vi "Lidar Motor Controler.vi"() -> ()   [LabVIEW 2009]
uses:
  Motor Output Global.vi
  Motor Control Global.vi
panel:
  out "number":fxp<+/-,18,1> format="%.18g"
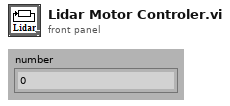
[diagram p1: front panel]
types:
  T1 = typedef "Strict Lidar Motor Control Cluster.ctl" = cluster{"Reset Encoder":bool, "Motor Enable":bool, "Choice of Control Type":enum32{"Direct Voltage Control", "Proportional Control", "PI Control", "Custom Compensator", "PID Control", "II-PID-DD Control"}, "Choice of Oscillation":enum32{"Oscillate Voltage", "Oscillate Setpoint", "No Oscillation"}, "Choice of Compensation":enum32{"None", "Computed Torque", "Mechanical Advantage", "CT & MA "}, "Choice of Error":enum32{"Gray Error", "Lidar Error", "Kent Error", "UberKent Error"}, "Units of pi rad 18b (s-fxp-1)":cluster{"Phi_B Set Point (pi rad)":fxp<+/-,18,1>, "Phi_A Set Point (pi rad)":fxp<+/-,18,1>, "Phi_Lidar Set Point (pi rad)":fxp<+/-,18,1>, "Phi_Lidar - Phi_A":fxp<+/-,18,1>, "Phi_mass-Phi_Lidar":fxp<+/-,18,1>, "Convert (enc) to (pi rad)":fxp<+/-,18,1>, "Oscillation Frequency (pi rad per 100KHz)":fxp<+/-,18,1>}, "Units of 18b (s-fxp-1) gain":cluster{"Proportional Gain":fxp<+/-,18,1>, " Integral Gain":fxp<+/-,18,1>, "Oscillation Setpoint Amplitude":fxp<+/-,18,1>, "Gravity Compensation Gain":fxp<+/-,18,1>, "Phi_B Set Point (enc) pre-gain":fxp<+/-,18,1>, "Phi_B Set Point (pi rad) pre-gain":fxp<+/-,18,1>, "Phi_A Set Point (pi rad) pre-gain":fxp<+/-,18,1>, "Phi_Lidar Set Point (pi rad) pre-gain":fxp<+/-,18,1>, "Derivative Gain":fxp<+/-,18,1>, "Double Integral Gain":fxp<+/-,18,1>, "Second Derivative Gain":fxp<+/-,18,1>}, "Units of 20b s-fxp-5 Voltage":cluster{"Oscillation Voltage Amplitude":fxp<+/-,20,5>, "Motor Voltage":fxp<+/-,20,5>}, "Units of encoder 32b uint":cluster{"Phi_B Set Point (enc)":i32, "Lidar Encoder Cap":i32}, "Debug Args":bool[], "Units of 8b int gain exponents":cluster{"Proportional Gain":i8, " Integral Gain":i8, "Oscillation Setpoint Amplitude":i8, "Gravity Compensation Gain":i8, "Phi_B Set Point (enc) pre-gain":i8, "Phi_B Set Point (pi rad) pre-gain":i8, "Phi_A Set Point (pi rad) pre-gain":i8, "Phi_Lidar Set Point (pi rad) pre-gain":i8, "Derivative Gain":i8, "Double Integral Gain":i8, "Second Derivative Gain":i8}}
  T2 = cluster{"Debug Args[0]":bool, "Debug Args[1]":bool, "Debug Args[2]":bool, "Debug Args[3]":bool, "Debug Args[4]":bool, "Debug Args[5]":bool, "Debug Args[6]":bool, "Debug Args[7]":bool, "Debug Args[8]":bool}
  T3 = typedef "Strict Lidar Motor Indicator Cluster.ctl" = cluster{"Phi_A":fxp<+/-,18,1>, "Phi_B":fxp<+/-,18,1>, "Output Voltage":fxp<+/-,20,5>, "Phi_Lidar":fxp<+/-,18,1>, "Phi_Mass":fxp<+/-,18,1>, "MA":fxp<+/-,18,1>, "Base Output":fxp<+/-,18,1>, "Error":fxp<+/-,18,1>, "Low Enc":i32, "High Enc":i32}
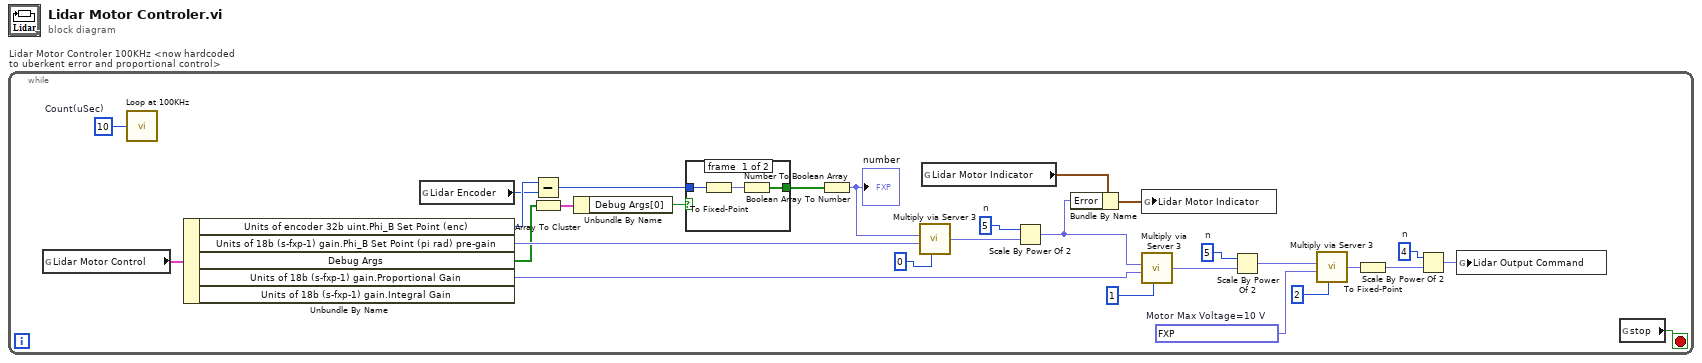
[diagram p0: block diagram]
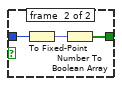
[diagram p2: hidden frame]
diagram:
  n1 = while "Lidar Motor Controler 100KHz <now hardcoded to uberkent error and proportional control>" {
    stop <- w29 stop-if-true
    w2 = 4  # n
    w5 = fxp<+/-,18,1> 0.625  # Motor Max Voltage=10 V
    w13 = 5  # n
    w14 = 5  # n
    w28 = u32 10  # Count(uSec)
    n2 = global read "Motor Control Global.vi" "Lidar Motor Control"() -> (w23:T1)
    n3 = call "Loop at 100KHz"("Count(uSec)"=w28) -> ()  [unwired: 1 out]
    n4 = Unbundle By Name(w23) -> ("Units of encoder 32b uint.Phi_B Set Point (enc)"=w22:i32, "Units of 18b (s-fxp-1) gain.Phi_B Set Point (pi rad) pre-gain"=w20:fxp<+/-,18,1>, "Debug Args"=w19:bool[], "Units of 18b (s-fxp-1) gain.Proportional Gain"=w16:fxp<+/-,18,1>)  [unwired: 1 out]
    n5 = global read "Motor Control Global.vi" "Lidar Encoder"() -> (w21:i32)
    n6 = Subtract(x=w22, y=w21) -> (x-y=w8:i32)
    n7 = Array To Cluster(array=w19) -> (cluster=w18:T2)
    n8 = Unbundle By Name(w18) -> ("Debug Args[0]"=w17:bool)
    n9 = case shown="True" w17 {
      tunnel: [w31 w35] -> w27
      tunnel: w8 -> [w30 w33]
      frame #0 {
        n10 = To Fixed-Point(number=w30) -> (fixed-point=w32:fxp<+/-,18,18>)  [unwired: 1 in]
        n11 = Number To Boolean Array(number=w32) -> (Boolean array=w31:bool[])
      }
      frame #1 {
        n12 = To Fixed-Point(number=w33) -> (fixed-point=w34:fxp<+/-,18,22>)  [unwired: 1 in]
        n13 = Number To Boolean Array(number=w34) -> (Boolean array=w35:bool[])
      }
    }
    n14 = Boolean Array To Number(Boolean array=w27) -> (number=w25:fxp<+/-,18,1>)
    "number" <- w25
    n15 = call "Multiply via Server 3.vi"("Unique 8b identifier"=u8 0, "Input B"=w20, "Input A"=w25) -> ("Output"=w15:fxp<+/-,18,1>)  [unwired: 3 in]
    n16 = global read "Motor Control Global.vi" "Lidar Motor Indicator"() -> (w11:T3)
    n17 = Scale By Power Of 2(n=w14, x=w15) -> (x*2^n=w9:fxp<+/-,18,1>)
    n18 = Bundle By Name(cluster=w11, "Error"=w9) -> (w10:T3)
    n19 = global write "Motor Control Global.vi" "Lidar Motor Indicator"(w10) -> ()
    n20 = call "Multiply via Server 3.vi"("Unique 8b identifier"=u8 1, "Input B"=w16, "Input A"=w9) -> ("Output"=w12:fxp<+/-,18,1>)  [unwired: 3 in]
    n21 = Scale By Power Of 2(n=w13, x=w12) -> (x*2^n=w6:fxp<+/-,18,1>)
    n22 = call "Multiply via Server 3.vi"("Unique 8b identifier"=u8 2, "Input B"=w5, "Input A"=w6) -> ("Output"=w4:fxp<+/-,18,1>)  [unwired: 3 in]
    n23 = To Fixed-Point(number=w4) -> (fixed-point=w3:fxp<+/-,20,5>)  [unwired: 1 in]
    n24 = Scale By Power Of 2(n=w2, x=w3) -> (x*2^n=w1:fxp<+/-,20,5>)
    n25 = global write "Motor Output Global.vi" "Lidar Output Command"(w1) -> ()
    n26 = global read "Motor Control Global.vi" "stop"() -> (w29:bool)
  }
